vi "数字处理.vi"() -> ()   [LabVIEW 2014]
uses:
  <vilib>/Analysis/NI_AALBase.lvlib
panel:
  out "标准差":dbl
  out "中值":dbl
  out "均方根":dbl
  out "算术平均":dbl
  out "波形图 2":dynamicdata(graph)
  out "波形图":dbl[](graph)
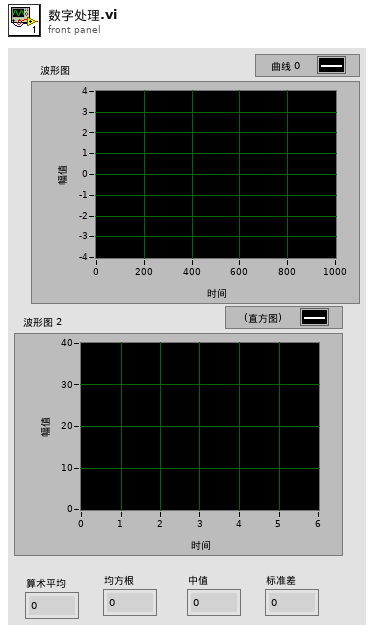
[diagram p1: front panel]
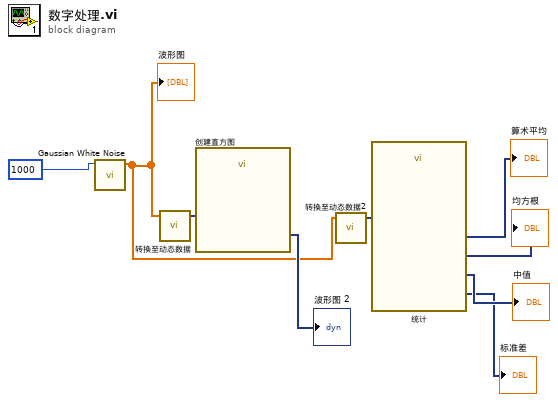
[diagram p0: block diagram]
diagram:
  n1 = call <vilib>:"Gaussian White Noise.vi"("samples"=1000) -> ("Gaussian noise pattern"=w5:dbl[])  [unwired: 9 in, 1 out]
  "波形图" <- w5
  n2 = call "转换至动态数据"("Array"=w5) -> ("Dynamic Data Type"=w8:dynamicdata)  [unwired: 3 in]
  n3 = call "创建直方图"("Signal"=w8) -> ("Histogram"=→"波形图 2":dynamicdata)  [unwired: 9 in, 1 out]
  n4 = call "转换至动态数据2"("Array"=w5) -> ("Dynamic Data Type"=w7:dynamicdata)  [unwired: 3 in]
  n5 = call "统计"("Signals"=w7) -> ("Median"=→"中值":dynamicdata, "Standard Dev"=→"标准差":dynamicdata, "RMS"=→"均方根":dynamicdata, "Arithmetic Mean"=→"算术平均":dynamicdata)  [unwired: 22 in, 1 out]
